vi "Determine Consecutive L-STF Peak Count.vi"(5 "reset peak count":bool, 7 "maximum peak index derivation":u8, 9 "peak index valid":bool, 10 "peak index":u16) -> (0 "output valid":bool, 1 "last peak index":u16, 2 "number of consecutive peaks":u8)   [LabVIEW 2020]
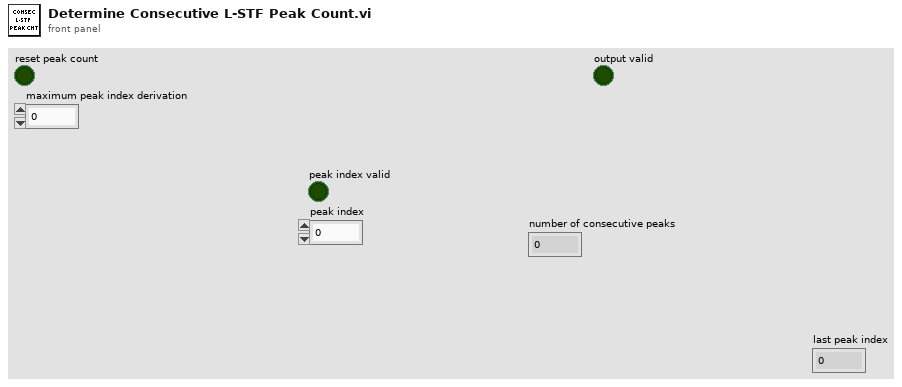
[diagram p1: front panel]
types:
  T1 = cluster{"EIFS":u32, "ACK timeout":u32, "CTS timeout":u32, "aRxPHYStartDelay":u32, "Frame control field length":u16, "Duration/ID field length":u16, "aSlotTime":u32, "aSIFSTime":u32, "PIFS":u32, "DIFS":u32, "Address field length":u16, "Sequence control field length":u16, "QoS control field length":u16, "HT control field length":u16, "FCS field length":u16, "MPDU delimiter length":u16, "MPDU delimiter signature":u16, "Max MPDU buffer length":u16, "timestamp steps / mks":u32, "L-STF periods / L-STF":u8, "sample / L-STF period":u8, "T_SIGNAL":u16, "N_tail":u16, "N_service":u16, "N_ES":u16, "N_SS":u16, "m_STBC":u16, "T_VHTSIGB":u16, "T_VHTPREAMBLE":u16, "T_VHTSIGA":u16, "T_LSIG":u16, "T_LEGPREAMBLE":u16, "NOFDM_VHTSIGB":u16, "T_SYM":u16, "T_SYML":u16, "NOFDM_PREAMBLE":u16, "NOFDM_SIGNAL":u16, "T_PREAMBLE":u16, "NOFDM_LEGPREAMBLE":u16, "NOFDM_VHTPREAMBLE":u16, "NOFDM_VHTSIGA":u16, "NOFDM_LSIG":u16, "NOFDM_VHTPREAMBLE 2":u16, "NOFDM_LSIG 2":u16}
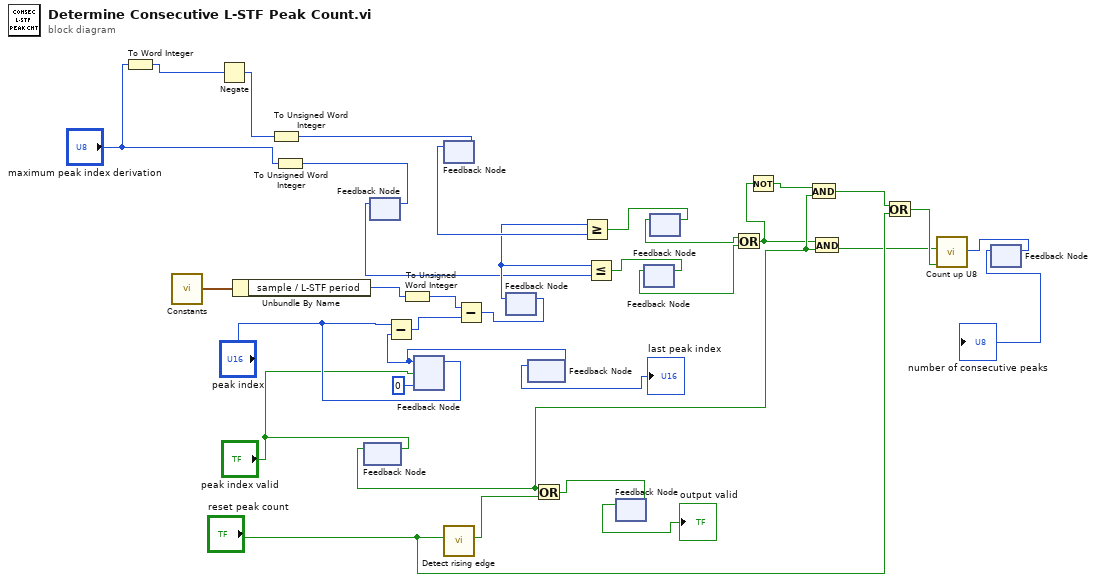
[diagram p0: block diagram]
diagram:
  n1 = To Word Integer(number="maximum peak index derivation") -> (16bit integer=w17:i16)
  n2 = call "Constants.vi"() -> ("output cluster"=w34:T1)  [unwired: 11 in]
  n3 = Negate(x=w17) -> (-x=w18:i16)
  n4 = Unbundle By Name(w34) -> ("sample / L-STF period"=w33:u8)
  n5 = To Unsigned Word Integer(number=w18) -> (unsigned 16bit integer=w20:u16)
  n6 = To Unsigned Word Integer(number="maximum peak index derivation") -> (unsigned 16bit integer=w19:u16)
  n7 = feedback #1() -> (w12:bool)  [unwired: 1 in]
  n8 = feedback-in #1("peak index valid") -> ()
  n9 = feedback #2() -> (w2:u16)  [unwired: 1 in]
  n10 = feedback-in #2(w19) -> ()
  n11 = To Unsigned Word Integer(number=w33) -> (unsigned 16bit integer=w32:u16)
  n12 = feedback-in #3("peak index", "peak index valid") -> ()
  n13 = feedback #3(u16 0 ("peak index")) -> (w29:u16)
  n14 = Subtract(x="peak index", y=w29) -> (x-y=w31:u16)
  n15 = feedback #4() -> (w21:u16)  [unwired: 1 in]
  n16 = feedback-in #4(w20) -> ()
  n17 = call "Detect rising edge.vi"("signal"="reset peak count") -> ("edge detected"=w23:bool)  [unwired: 10 in]
  n18 = Subtract(x=w32, y=w31) -> (x-y=w22:u16)
  n19 = feedback #5() -> (w3:u16)  [unwired: 1 in]
  n20 = feedback-in #5(w22) -> ()
  n21 = feedback #6() -> (→"last peak index":u16)  [unwired: 1 in]
  n22 = feedback-in #6(w29) -> ()
  n23 = Or(x=w12, y=w23) -> (x .or. y?=w24:bool)
  n24 = Greater Or Equal?(x=w3, y=w21) -> (x >= y?=w15:bool)
  n25 = Less Or Equal?(x=w3, y=w2) -> (x <= y?=w1:bool)
  n26 = feedback-in #7(w24) -> ()
  n27 = feedback #7() -> (→"output valid":bool)  [unwired: 1 in]
  n28 = feedback #8() -> (w13:bool)  [unwired: 1 in]
  n29 = feedback-in #8(w1) -> ()
  n30 = feedback #9() -> (w14:bool)  [unwired: 1 in]
  n31 = feedback-in #9(w15) -> ()
  n32 = Or(x=w14, y=w13) -> (x .or. y?=w10:bool)
  n33 = Not(x=w10) -> (.not. x?=w11:bool)
  n34 = And(x=w11, y=w12) -> (x .and. y?=w8:bool)
  n35 = And(x=w10, y=w12) -> (x .and. y?=w6:bool)
  n36 = Or(x=w8, y="reset peak count") -> (x .or. y?=w7:bool)
  n37 = call "Count up U8.vi"("reset"=w7, "increment"=w6) -> ("count out"=w5:u8)  [unwired: 9 in]
  n38 = feedback #10() -> (→"number of consecutive peaks":u8)  [unwired: 1 in]
  n39 = feedback-in #10(w5) -> ()
